vi "Initialise Light.vi"(8 "error in (no error)":errorcluster, 10 "Resource Directory":path, 11 "Scene in":refnum<class "Scene.lvclass">) -> (0 "error out":errorcluster, 3 "Scene out":refnum<class "Scene.lvclass">)   [LabVIEW 2020, in "Application.lvlib" / "Scene.lvclass"]
uses:
  Scene.lvclass
  Scene.lvclass/Scene.ctl
  FPGA/Libraries/3D/3D (FPGA).lvlib
  FPGA/Libraries/3D/Vector 3D.ctl
  FPGA/Libraries/3D/Transform.ctl
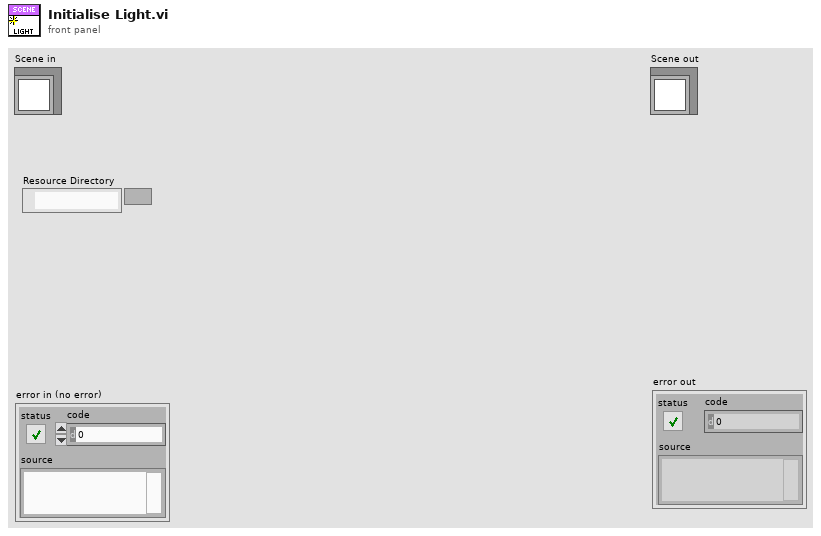
[diagram p1: front panel]
types:
  T1 = typedef "3D (FPGA).lvlib/Transform.ctl" = cluster{"Position":T2, "Rotation":T2, "Scale":T2}
  T2 = typedef "3D (FPGA).lvlib/Vector 3D.ctl" = cluster{"x":sgl, "y":sgl, "z":sgl}
  T3 = typedef "3D (FPGA).lvlib/Object.ctl" = cluster{"Triangles":T4[], "Transform":T1, "Name":string, "Alpha Blending Enabled":bool, "Alpha":dbl, "Turntable Enabled":bool, "Material":T7}
  T4 = typedef "3D (FPGA).lvlib/Triangle.ctl" = cluster{"Vertex 1":T5, "Vertex 2":T5, "Vertex 3":T5, "Alpha":dbl, "Alpha Blending Enabled":bool, "Colour":u32, "Material":T7}
  T5 = typedef "3D (FPGA).lvlib/Vertex.ctl" = cluster{"Position":T2, "UV":T6, "Colour":u32}
  T6 = typedef "Raster (FPGA).lvlib/UV.ctl" = cluster{"u":sgl, "v":sgl}
  T7 = typedef "3D (FPGA).lvlib/Material.ctl" = cluster{"Diffuse Colour":u32, "Texture":T8}
  T8 = typedef "Raster (FPGA).lvlib/Texture.ctl" = cluster{"Pixels":refnum<data-value>, "Size":T9}
  T9 = typedef "Raster (FPGA).lvlib/Rectangle Dimensions.ctl" = cluster{"Width":u32, "Height":u32}
  T10 = cluster{"Position":cluster{"x":dbl, "y":dbl, "z":dbl}, "UV":cluster{"u":dbl, "v":dbl}, "Colour":dbl}
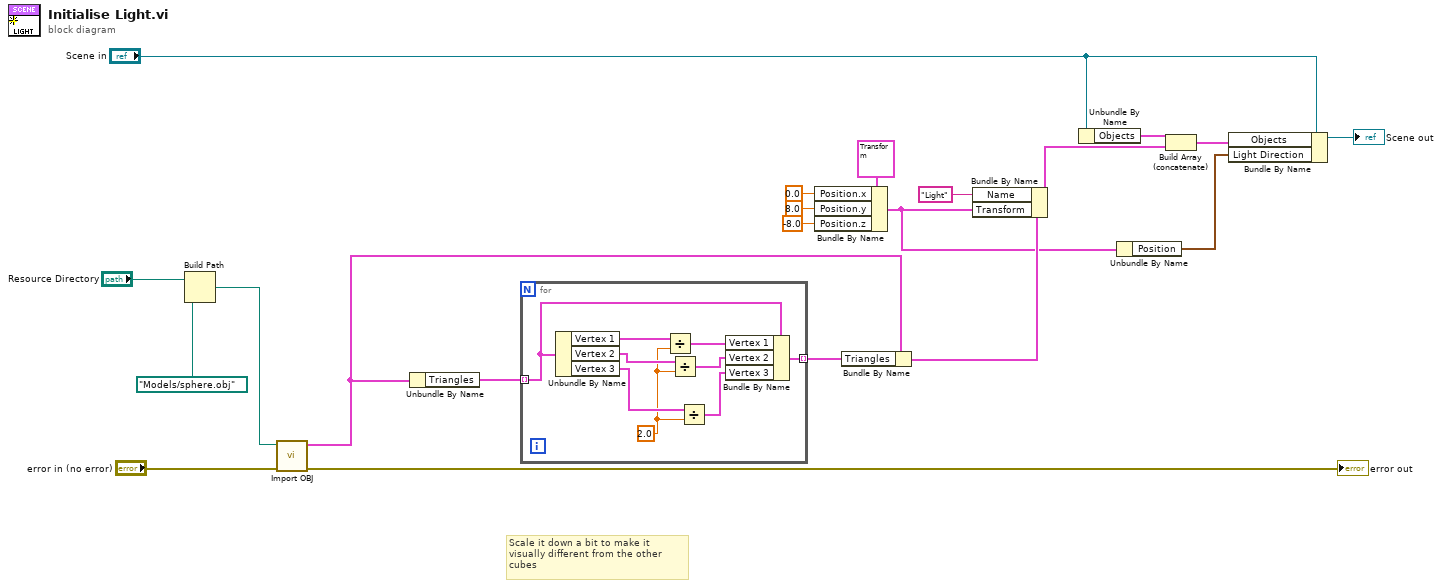
[diagram p0: block diagram]
diagram:
  # "Scale it down a bit to make it visually different from the other cubes"
  n1 = Build Path(base path="Resource Directory", name or relative path=path "Models/sphere.obj") -> (appended path=w20:path)
  n2 = call "Import OBJ.vi"("error in (no error)"="error in (no error)", "Object"=w20) -> ("error out"=→"error out":errorcluster, "Object"=w7:T3)  [unwired: 8 in]
  n3 = Unbundle By Name(w7) -> ("Triangles"=w1:T4[])
  n4 = for {
    tunnel: [w28] -> w5 mode=indexing
    tunnel: w1 -> [w29] mode=indexing
    w22 = 2.0
    n5 = Unbundle By Name(w29) -> ("Vertex 1"=w30:T5, "Vertex 2"=w27:T5, "Vertex 3"=w23:T5)
    n6 = Divide(x=w30, y=w22) -> (x/y=w26:T10)
    n7 = Divide(x=w27, y=w22) -> (x/y=w25:T10)
    n8 = Divide(x=w23, y=w22) -> (x/y=w24:T10)
    n9 = Bundle By Name(cluster=w29, "Vertex 1"=w26, "Vertex 2"=w25, "Vertex 3"=w24) -> (w28:T4)
  }
  n10 = Bundle By Name(cluster=T1 {"Position"={"x"=2.0, "y"=1.0, "z"=-5.0}, "Rotation"={"x"=0.0, "y"=0.0, "z"=0.0}, "Scale"={"x"=0.0, "y"=0.0, "z"=0.0}} ("Transform"), "Position.x"=sgl 0.0, "Position.y"=sgl 8.0, "Position.z"=sgl -8.0) -> (w3:T1)
  n11 = Bundle By Name(cluster=w7, "Triangles"=w5) -> (w6:T3)
  n12 = Bundle By Name(cluster=w6, "Name"="Light", "Transform"=w3) -> (w8:T3)
  n13 = Unbundle By Name("Scene in") -> ("Objects"=w13:T3[])
  n14 = Unbundle By Name(w3) -> ("Position"=w2:T2)
  n15 = Build Array (concatenate)(w13, w8) -> (w4:T3[])
  n16 = Bundle By Name(cluster="Scene in", "Objects"=w4, "Light Direction"=w2) -> (→"Scene out":refnum<class "Scene.lvclass">)
